vi "Frequency Response Function (Real-Im) N-1.vi"(0 "time signals X":waveform(dbl)[](array[waveform]), 1 "restart averaging (F)":bool, 2 "window parameter":dbl=nan, 5 "time signal Y":waveform(dbl), 7 "window":T1=1 items=["Rectangle"=0, "Hanning"=1, "Hamming"=2, "Blackman-Harris"=3, "Exact Blackman"=4, "Blackman"=5, "Flat Top"=6, "4 Term B-Harris "=7, "7 Term B-Harris"=8, "Low Sidelobe"=9, "Blackman Nuttall"=11, "Triangle"=30, "Bartlett-Hanning"=31, "Bohman"=32, "Parzen"=33, "Welch"=34, "Kaiser"=60, "Dolph-Chebyshev"=61, "Gaussian"=62], 11 "error in (no error)":errorcluster, 12 "averaging parameters":T2={"averaging mode"=enum."No averaging", "weighting mode"=enum."Exponential", "number of averages"=10} {"number of averages" min=1}, 13 "FRF Mode":enum16{"H1", "H2", "H3"}(ring)) -> (3 "averaging done":bool, 4 "real parts":cluster{"f0":dbl, "df":dbl, "real part":dbl[]}[](array[cluster]) {"real part" format="%.2p"; "f0" format="%0.2p"; "df" format="%0.2p"}, 6 "imaginary parts":cluster{"f0":dbl, "df":dbl, "imag part":dbl[]}[](array[cluster]) {"imag part" format="%.2p"; "f0" format="%0.2p"; "df" format="%0.2p"}, 8 "coherences":cluster{"f0":dbl, "df":dbl, "coherence":dbl[]}[](array[cluster]) {"coherence" format="%.2g"; "df" format="%.2p"; "f0" format="%.2p"}, 10 "averages completed":dbl format="%.2p", 15 "error out":errorcluster)   [LabVIEW 2020, in "NI_MAPro.lvlib"]
doc: "Computes the frequency response and the coherence based on the input signals. Results are returned as <B>real part</B>, <B>imaginary part</B>, and <B>coherence</B>."
uses:
  NI_MAPro.lvlib
  windowTd.ctl
  2-chan State.ctl
  NI_MABase.lvlib
  NI_AALPro.lvlib
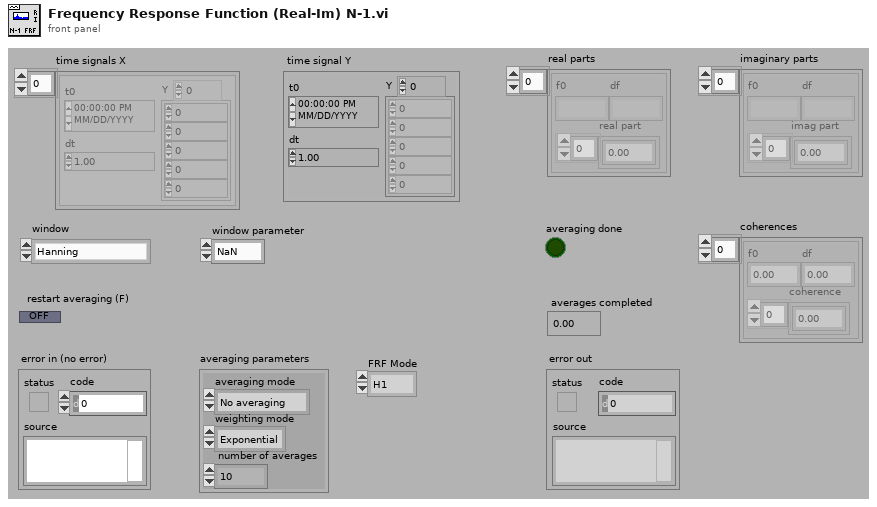
[diagram p1: front panel]
types:
  T1 = typedef "NI_AALPro.lvlib/windowTd.ctl" = u32
  T2 = cluster{"averaging mode":enum16{"No averaging", "Vector averaging", "RMS averaging", "Peak hold"}, "weighting mode":enum16{"Linear", "Exponential"}, "number of averages":u32}
  T3 = typedef "NI_MAPro.lvlib/2-chan State.ctl" = cluster{"Sx":cdb[], "Sy":cdb[], "Sxx":dbl[], "Syy":dbl[], "Sxy":cdb[], "block size":i32, "df":dbl, "dt":dbl, "avgs completed":dbl, "spectrum parameters":cluster{"averaging parameters":cluster{"averaging mode":enum16{"No averaging", "Vector averaging", "RMS averaging", "Peak hold"}, "weighting mode":enum16{"Linear", "Exponential"}, "number of averages":u32}, "window":T1}, "lin avg done":bool, "t0 history":dbl, "dt history":dbl, "timestamp":dbl}
  T4 = cluster{"f0":dbl, "df":dbl, "imag or phase":dbl[]}
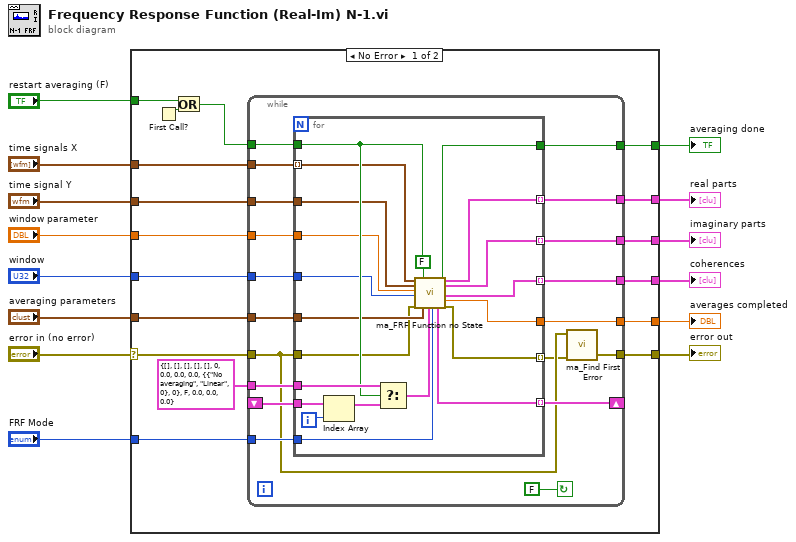
[diagram p0: block diagram]
diagram:
  n1 = case shown="No Error" "error in (no error)" {
    selector: "error in (no error)" -> [w28 w72]
    tunnel: [w27 w72] -> w13
    tunnel: "restart averaging (F)" -> [w26 _]
    tunnel: "time signals X" -> [w25 _]
    tunnel: "time signal Y" -> [w24 _]
    tunnel: "window" -> [w23 _]
    tunnel: "window parameter" -> [w22 _]
    tunnel: "averaging parameters" -> [w21 _]
    tunnel: "FRF Mode" -> [w20 _]
    tunnel: [w19 _] -> w5
    tunnel: [w18 _] -> w4
    tunnel: [w17 _] -> w3
    tunnel: [w16 _] -> w2
    tunnel: [w15 _] -> w1
    frame No Error {
      n2 = First Call?() -> (First Call?: T/F=w31:bool)
      n3 = Or(x=w26, y=w31) -> (x .or. y?=w29:bool)
      n4 = while {
        tunnel: T3 {"Sx"=[], "Sy"=[], "Sxx"=[], "Syy"=[], "Sxy"=[], "block size"=0, "df"=0.0, "dt"=0.0, "avgs completed"=0.0, "spectrum parameters"={"averaging parameters"={"averaging mode"=enum."No averaging", "weighting mode"=enum."Linear", "number of averages"=0}, "window"=0}, "lin avg done"=FALSE, "t0 history"=0.0, "dt history"=0.0, "timestamp"=0.0} ("state info out") -> [w50]
        tunnel: w29 -> [w49]
        tunnel: w25 -> [w48]
        tunnel: w24 -> [w47]
        tunnel: w23 -> [w46]
        tunnel: w21 -> [w45]
        tunnel: w20 -> [w44]
        tunnel: [w43] -> w19
        tunnel: [w42] -> w15
        tunnel: w28 -> [w35]
        tunnel: [w41] -> w18
        tunnel: [w40] -> w17
        tunnel: [w39] -> w16
        shift-right: [w37] -> _
        shift-left: _ -> [w36]
        tunnel: [w33] -> w27
        tunnel: w22 -> [w32]
        stop <- FALSE continue-if-true
        n5 = for {
          tunnel: w49 -> [w64]
          tunnel: [w71] -> w43
          tunnel: [w70] -> w42
          tunnel: [w69] -> w41 mode=indexing
          tunnel: [w66] -> w40 mode=indexing
          tunnel: w50 -> [w65]
          tunnel: w48 -> [w63] mode=indexing
          tunnel: w47 -> [w57]
          tunnel: w46 -> [w62]
          tunnel: w45 -> [w61]
          tunnel: w44 -> [w60]
          tunnel: [w59] -> w39 mode=indexing
          tunnel: w35 -> [w58]
          tunnel: [w56] -> w37 mode=indexing
          tunnel: w36 -> [w54]
          tunnel: [w52] -> w34 mode=indexing
          tunnel: w32 -> [w51]
          i -> [w55]
          n6 = Index Array(array=w54, index=w55) -> (element=w53:T3)
          n7 = Select(t=w65, s=w64, f=w53) -> (s? t:f=w68:T3)
          n8 = call "ma_FRF Function no State.vi"("time signal X"=w63, "time signal Y"=w57, "window parameter"=w51, "window"=w62, "error in (no error)"=w58, "restart averaging (F)"=w64, "averaging parameters"=w61, "mag-phase"=FALSE, "state info"=w68, "FRF Mode"=w60) -> ("averaging done"=w71:bool, "state info out"=w56:T3, "real or mag"=w69:cluster{"f0":dbl, "df":dbl, "real or mag":dbl[]}, "imag or phase"=w66:T4, "coherence"=w59:cluster{"f0":dbl, "df":dbl, "coherence":dbl[]}, "averages completed"=w70:dbl, "error out"=w52:errorcluster)  [unwired: 1 in, 2 out]
        }
        n9 = call "ma_Find First Error.vi"("error array in"=w34, "error in 1 (no error)"=w35) -> ("error out"=w33:errorcluster)  [unwired: 2 in, 3 out]
      }
    }
    frame Error {
    }
  }
  "error out" <- w13
  "averages completed" <- w1
  "averaging done" <- w5
  "coherences" <- w2
  "real parts" <- w4
  "imaginary parts" <- w3
